vi "sub_getQueueElements.vi"(11 "Q1":refnum<queue>) -> ()   [LabVIEW 2018]
uses:
  guess.ctl
panel:
  out "elements":T1[](array[typedef])
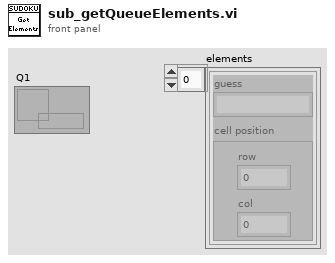
[diagram p1: front panel]
types:
  T1 = typedef "guess.ctl" = cluster{"cell position":cluster{"row":i32, "col":i32}, "guess":string}
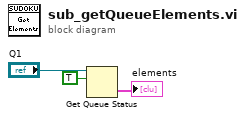
[diagram p0: block diagram]
diagram:
  n1 = Get Queue Status(queue="Q1", return elements? (F)=TRUE) -> (elements=→"elements":T1[])  [unwired: 1 in, 7 out]
